vi "Init Loop Data.vi"(5 "State Control":T1, 7 "VolatusAPI":refnum<class "VolatusAPI.lvclass">, 8 "MultiErrors":refnum<class "MultiErrors.lvclass">, 9 "State":T10, 10 "Sequencer":refnum<class "MessageQ.lvclass">, 11 "State in":refnum<class "State.lvclass">) -> (0 "error out":refnum<class "MultiErrors.lvclass">, 2 "State Loop Data":T2, 3 "State out":refnum<class "State.lvclass">)   [LabVIEW 2023, in "VolatusSeq.lvlib" / "State.lvclass"]
uses:
  State.lvclass
  VolatusErrorUtilities/MultiErrors/MultiErrors.lvclass
  VolatusSeqConfig/State.ctl
  VolatusSeqConfig/Step.ctl
  State Loop Data.ctl
  Iteration Actions/Iteration Actions.lvclass
  Variables/Variables.lvclass
  Command.ctl
  VolatusSeqConfig/Command Type.ctl
  messages/CmdDigital/Data.ctl
  messages/CmdAnalog/Data.ctl
  Send Type.ctl
  Sequence Time.ctl
  Volatus/VolatusAPI/VolatusAPI.lvclass
  State Control.ctl
  State.lvclass/State.ctl
  VolatusErrorUtilities/MultiErrors/MultiErrors.lvclass/MultiErrors.ctl
  Transition/Transition.lvclass
  VolatusSeq.lvlib
  Volatus/MessageQ/MessageQ.lvclass
  VolatusSeqConfig/VolatusSeqConfig.lvlib
  messages/CmdAnalog/CmdAnalog.lvlib
  messages/CmdDigital/CmdDigital.lvlib
  lv-vecto/Vecto/Channel DBL/Channel DBL.lvclass
  Format String/Format String.lvclass
  VolatusSeqConfig/Debug Flags.ctl
  VolatusSeqConfig/Command Config/Command Config.lvclass
  VolatusSeqConfig/Transition Config/Transition Config.lvclass
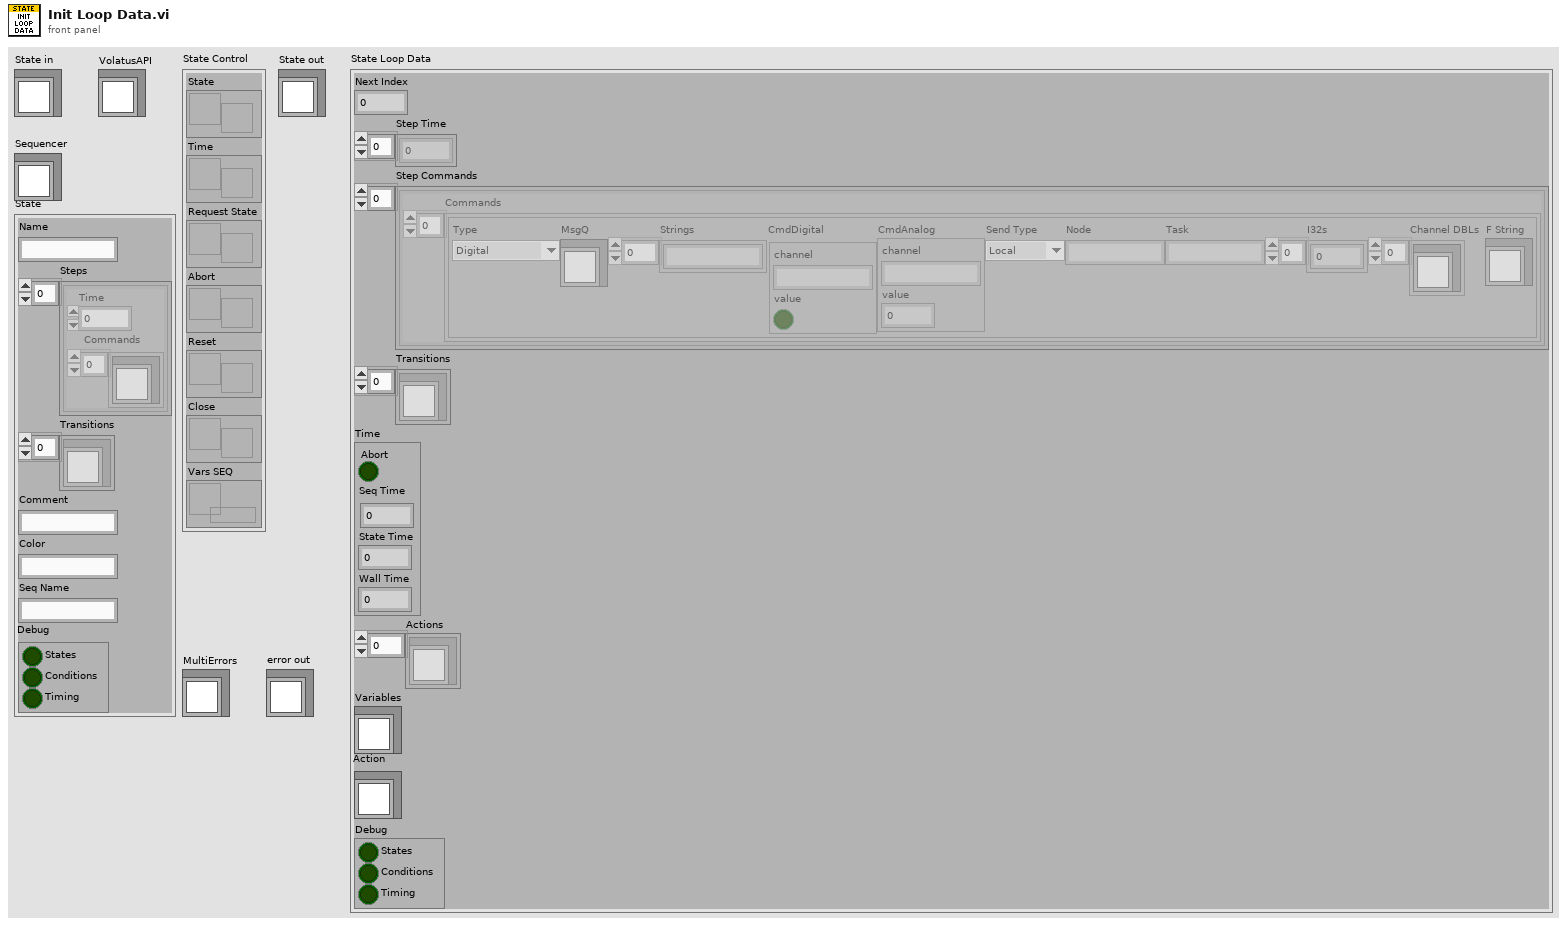
[diagram p1: front panel]
types:
  T1 = typedef "VolatusSeq.lvlib/State Control.ctl" = cluster{"State":refnum<notifier>, "Time":refnum<notifier>, "Request State":refnum<notifier>, "Abort":refnum<notifier>, "Reset":refnum<notifier>, "Close":refnum<notifier>, "Vars SEQ":refnum<queue>}
  T2 = typedef "VolatusSeq.lvlib/State.lvclass/State Loop Data.ctl" = cluster{"Next Index":i32, "Step Time":dbl[], "Step Commands":cluster{"Commands":T3[]}[], "Transitions":refnum<class "Transition.lvclass">[], "Time":T8, "Actions":refnum<class "Iteration Actions.lvclass">[], "Variables":refnum<class "Variables.lvclass">, "Action":refnum<class "Iteration Actions.lvclass">, "Debug":T9}
  T3 = typedef "VolatusSeq.lvlib/Command.ctl" = cluster{"Type":T4, "MsgQ":refnum<class "MessageQ.lvclass">, "Strings":string[], "CmdDigital":T5, "CmdAnalog":T6, "Send Type":T7, "Node":string, "Task":string, "I32s":i32[], "Channel DBLs":refnum<class "Channel DBL.lvclass">[], "F String":refnum<class "Format String.lvclass">}
  T4 = typedef "VolatusSeqConfig.lvlib/Command Type.ctl" = enum16{"Digital", "Numeric", "Transition", "Stop", "StartLog", "StopLog", "Start", "Event", "Error", "HTTP", "ResetVar", "IncVar", "DecVar", "SaveVar", "LoadVar", "AddVar", "SubVar", "SetVar", "AddToVar"}
  T5 = typedef "CmdDigital.lvlib/Data.ctl" = cluster{"channel":string, "value":bool}
  T6 = typedef "CmdAnalog.lvlib/Data.ctl" = cluster{"channel":string, "value":dbl}
  T7 = typedef "VolatusSeq.lvlib/Send Type.ctl" = enum16{"Local", "Remote"}
  T8 = typedef "VolatusSeq.lvlib/Sequence Time.ctl" = cluster{"Abort":bool, "Seq Time":dbl, "State Time":dbl, "Wall Time":dbl}
  T9 = typedef "VolatusSeqConfig.lvlib/Debug Flags.ctl" = cluster{"States":bool, "Conditions":bool, "Timing":bool}
  T10 = typedef "VolatusSeqConfig.lvlib/State.ctl" = cluster{"Name":string, "Steps":T11[], "Transitions":refnum<class "Transition Config.lvclass">[], "Comment":string, "Color":string, "Seq Name":string, "Debug":T9}
  T11 = typedef "VolatusSeqConfig.lvlib/Step.ctl" = cluster{"Time":dbl, "Commands":refnum<class "Command Config.lvclass">[]}
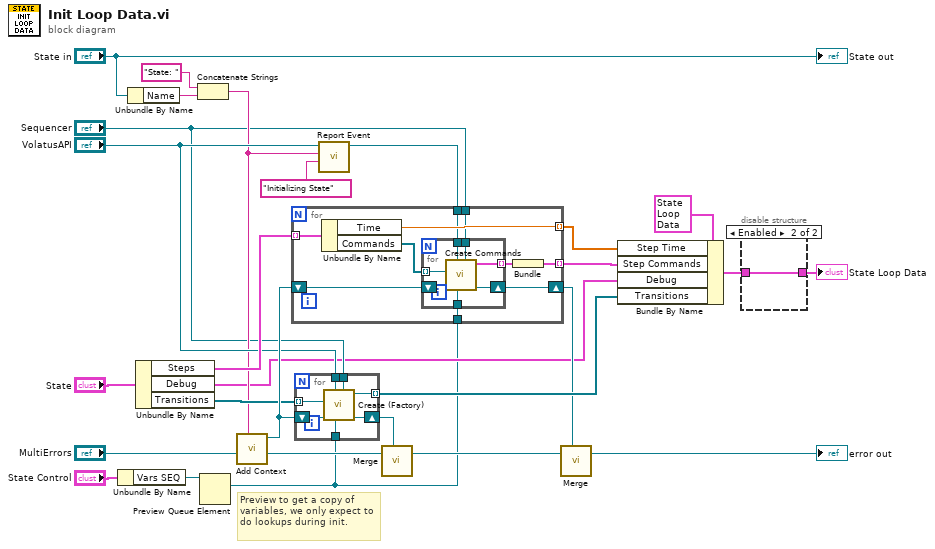
[diagram p0: block diagram]
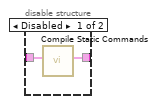
[diagram p2: hidden frame]
diagram:
  # "Preview to get a copy of variables, we only expect to do lookups during init."
  n1 = Unbundle By Name("State Control") -> ("Vars SEQ"=w2:refnum<queue>)
  n2 = Unbundle By Name("State in") -> ("Name"=w15:string)
  n3 = Unbundle By Name("State") -> ("Steps"=w26:T11[], "Debug"=w4:T9, "Transitions"=w21:refnum<class "Transition Config.lvclass">[])
  n4 = Concatenate Strings("State: ", w15) -> (w8:string)
  n5 = Preview Queue Element(queue=w2) -> (element=w1:refnum<class "Variables.lvclass">)  [unwired: 2 in, 3 out]
  n6 = call "Add Context.vi"("Context"=w8, "MultiErrors in"="MultiErrors") -> ("Original Context"=w12:refnum<class "MultiErrors.lvclass">, "Added Context"=w28:refnum<class "MultiErrors.lvclass">)  [unwired: 8 in]
  n7 = for {
    tunnel: w21 -> [w35] mode=indexing
    tunnel: [w34] -> w20 mode=indexing
    tunnel: "VolatusAPI" -> [w33]
    shift-right: [w31] -> w11
    shift-left: w28 -> [w32]
    tunnel: "Sequencer" -> [w30]
    tunnel: w1 -> [w29]
    n8 = call "Create (Factory).vi"("Sequencing"=w30, "Variables"=w29, "VolatusAPI"=w33, "MultiErrors"=w32, "Transition Config"=w35) -> ("MultiErrors out"=w31:refnum<class "MultiErrors.lvclass">, "Transition out"=w34:refnum<class "Transition.lvclass">)  [unwired: 5 in]
  }
  n9 = call "Report Event.vi"("Message"="Initializing State", "Context"=w8, "VolatusAPI in"="VolatusAPI") -> ("VolatusAPI out"=w9:refnum<class "VolatusAPI.lvclass">)  [unwired: 7 in, 1 out]
  n10 = for {
    tunnel: w26 -> [w45] mode=indexing
    tunnel: [w44] -> w24 mode=indexing
    tunnel: [w43] -> w23 mode=indexing
    tunnel: w9 -> [w41]
    shift-right: [w38] -> w10
    shift-left: w28 -> [w39]
    tunnel: "Sequencer" -> [w37]
    tunnel: w1 -> [w36]
    n11 = Unbundle By Name(w45) -> ("Time"=w44:dbl, "Commands"=w42:refnum<class "Command Config.lvclass">[])
    n12 = for {
      tunnel: w42 -> [w52] mode=indexing
      tunnel: w41 -> [w51]
      tunnel: [w50] -> w40 mode=indexing
      shift-right: [w48] -> w38
      shift-left: w39 -> [w49]
      tunnel: w37 -> [w47]
      tunnel: w36 -> [w46]
      n13 = call "Create Commands.vi"("Sequencer"=w47, "Variables"=w46, "VolatusAPI"=w51, "error in (no error)"=w49, "Command Config"=w52) -> ("error out"=w48:refnum<class "MultiErrors.lvclass">, "Command"=w50:T3)  [unwired: 5 in]
    }
    n14 = Bundle(w40) -> (w43:cluster{T3[]})  [unwired: 1 in]
  }
  n15 = call "Merge.vi"("First Error In"=w12, "Second Error In"=w11) -> ("MultiErrors out"=w13:refnum<class "MultiErrors.lvclass">)  [unwired: 5 in]
  n16 = call "Merge.vi"("First Error In"=w13, "Second Error In"=w10) -> ("MultiErrors out"=→"error out":refnum<class "MultiErrors.lvclass">)  [unwired: 5 in]
  n17 = Bundle By Name(cluster=T2 {"Next Index"=0, "Step Time"=[], "Step Commands"=[], "Transitions"=[], "Time"={"Abort"=FALSE, "Seq Time"=0.0, "State Time"=0.0, "Wall Time"=0.0}, "Actions"=[], "Variables"=refnum, "Action"=refnum, "Debug"={"States"=FALSE, "Conditions"=FALSE, "Timing"=FALSE}} ("State Loop Data"), "Step Time"=w24, "Step Commands"=w23, "Debug"=w4, "Transitions"=w20) -> (w22:T2)
  n18 = disable-structure shown="Enabled" {
    disable-tunnel: w22 -> [w54 w55]
    disable-tunnel: [w53 w55] -> w6
    frame Disabled {
      n19 = call "Compile Static Commands.vi"("State Loop Data in"=w54) -> ("State Loop Data out"=w53:T2)  [unwired: 10 in]
    }
    frame Enabled {
    }
  }
  "State Loop Data" <- w6
  "State out" <- "State in"
